vi "UI.LoadComboBoxes.vi"(8 "error in (no error)":errorcluster, 11 "State Variables":T1={"Aliases.All"=[], "Aliases.Outputs"=[], "UI.Sequence#ofColumns"=0, "SysDef.Path"=path "", "UI.SequenceRef"=refnum, "UI.StepInformationRef"=refnum, "UI.AbortRef"=refnum, "UI.GraphRef"=refnum, "UI.ViewRef"=refnum, "UI.IterationsRef"=refnum, "UI.IterationInformationRef"=refnum, "INI.Settings"={"Build Location"=path "C:/Simple Sequence Editor/SequenceRepo", "LoggingLocation"=path ""}, "NIVS.Workspace Event"=refnum, "UI.SkipChannel"=refnum, "NIVS.Launched?"=FALSE, "UI.DurationChannel"=refnum}) -> (0 "error out":errorcluster)   [LabVIEW 2015, in "Simple Sequence Tools - Editor.lvlib"]
uses:
  Simple Sequence Tools - Editor.lvlib
  Types/Main.StateVariables.ctl
  Shared/Types/Channel.Properties.ctl
  Shared/Types/INI.Settings
  Shared/Simple Sequence Tools - Shared.lvlib
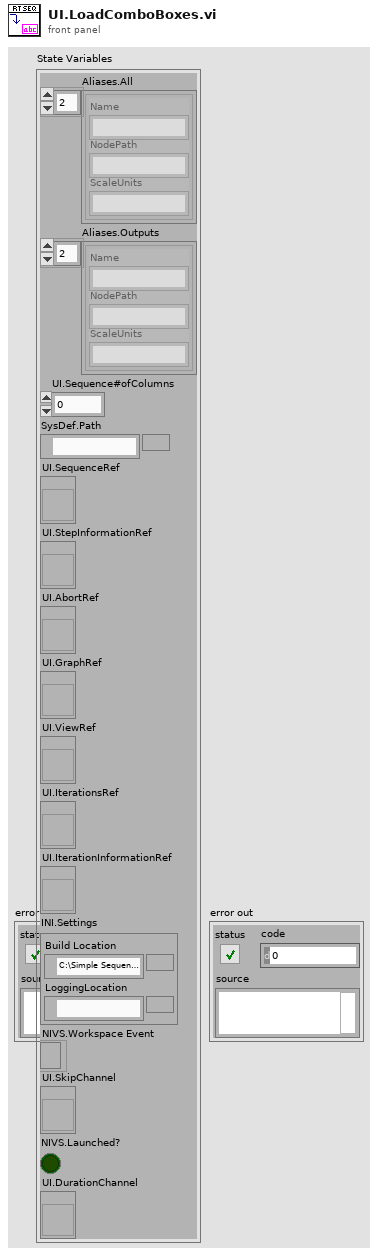
[diagram p1: front panel]
types:
  T1 = typedef "Simple Sequence Tools - Editor.lvlib/Main.StateVariables.ctl" = cluster{"Aliases.All":T2[], "Aliases.Outputs":T2[], "UI.Sequence#ofColumns":i32, "SysDef.Path":path, "UI.SequenceRef":refnum<vi>, "UI.StepInformationRef":refnum<vi>, "UI.AbortRef":refnum<vi>, "UI.GraphRef":refnum<vi>, "UI.ViewRef":refnum<vi>, "UI.IterationsRef":refnum<vi>, "UI.IterationInformationRef":refnum<vi>, "INI.Settings":T3, "NIVS.Workspace Event":refnum<event-registration>, "UI.SkipChannel":refnum<vi>, "NIVS.Launched?":bool, "UI.DurationChannel":refnum<vi>}
  T2 = typedef "Simple Sequence Tools - Shared.lvlib/Channel.Properties.ctl" = cluster{"Name":string, "NodePath":string, "ScaleUnits":string}
  T3 = typedef "Simple Sequence Tools - Shared.lvlib/INI.Settings" = cluster{"Build Location":path, "LoggingLocation":path}
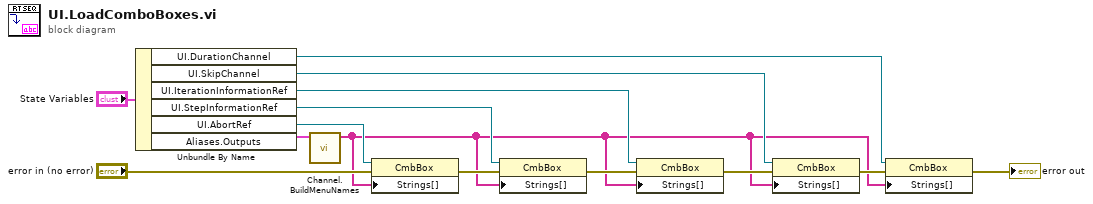
[diagram p0: block diagram]
diagram:
  n1 = Unbundle By Name("State Variables") -> ("UI.DurationChannel"=w1:refnum<vi>, "UI.SkipChannel"=w5:refnum<vi>, "UI.IterationInformationRef"=w13:refnum<vi>, "UI.StepInformationRef"=w11:refnum<vi>, "UI.AbortRef"=w9:refnum<vi>, "Aliases.Outputs"=w8:T2[])
  n2 = call "Channel.BuildMenuNames.vi"("Aliases"=w8) -> ("Aliases Array"=w2:string[])  [unwired: 10 in]
  n3 = property class="CmbBox"(reference=w9, error in="error in (no error)", "Strings[]"=w2) -> (error out=w10:errorcluster)  [unwired: 1 out]
  n4 = property class="CmbBox"(reference=w11, error in=w10, "Strings[]"=w2) -> (error out=w14:errorcluster)  [unwired: 1 out]
  n5 = property class="CmbBox"(reference=w13, error in=w14, "Strings[]"=w2) -> (error out=w6:errorcluster)  [unwired: 1 out]
  n6 = property class="CmbBox"(reference=w5, error in=w6, "Strings[]"=w2) -> (error out=w4:errorcluster)  [unwired: 1 out]
  n7 = property class="CmbBox"(reference=w1, error in=w4, "Strings[]"=w2) -> (error out=→"error out":errorcluster)  [unwired: 1 out]
